vi "Modify_Status.vi"(10 "Line 2":string, 11 "Line 1":string) -> (3 "resulting string":string)   [LabVIEW 2017]
doc: "Modificar mensaje que se muestra al usuario en la pantalla principal."
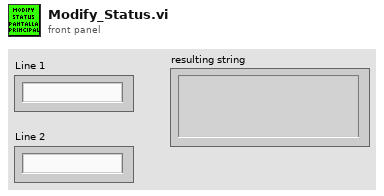
[diagram p1: front panel]
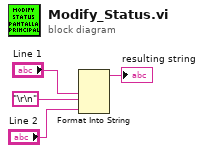
[diagram p0: block diagram]
diagram:
  n1 = Format Into String("Line 1", "\r\n", "Line 2") -> (resulting string=→"resulting string":string)  [unwired: 3 in, 1 out]
